vi "vdc_state_driver.vi"(1 "State Signal":dbl) -> (0 "VDC State":string)   [LabVIEW 2017]
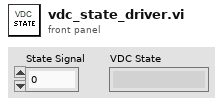
[diagram p1: front panel]
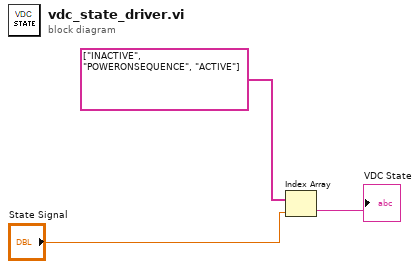
[diagram p0: block diagram]
diagram:
  n1 = Index Array(array=string[] ["INACTIVE", "POWERONSEQUENCE", "ACTIVE"], index="State Signal") -> (element=→"VDC State":string)
